vi "Actuator Calculations.vi"(9 "CV2 Flow Rate:":dbl, 10 "CV1 Flow Rate:":dbl) -> (1 "CV2 Voltage":dbl, 2 "CV1 Voltage":dbl)   [LabVIEW 2018]
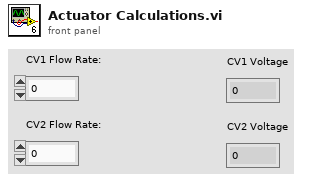
[diagram p1: front panel]
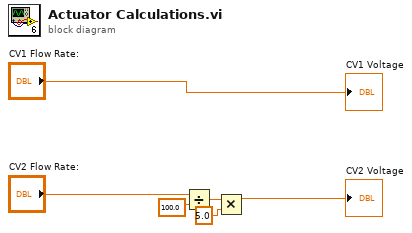
[diagram p0: block diagram]
diagram:
  n1 = Divide(x="CV2 Flow Rate:", y=100.0) -> (x/y=w6:dbl)
  n2 = Multiply(x=w6, y=5.0) -> (x*y=→"CV2 Voltage":dbl)
  "CV1 Voltage" <- "CV1 Flow Rate:"
